vi "Pre Launch Init.vi"(11 "VG-VNA_GUI in":refnum<class "VG-VNA_GUI.lvclass">) -> (0 "error out":errorcluster, 3 "VG-VNA_GUI out":refnum<class "VG-VNA_GUI.lvclass">)   [LabVIEW 2020, in "VG-VNA_GUI.lvlib" / "VG-VNA_GUI.lvclass"]
doc: "(<B>Filename</B>: Actor Framework.lvlib:Actor.lvclass:Pre Launch Init.vi)\n\nDefines behavior that occurs after the Launch Nested Actor method is invoked but before the actor's Actor Core method begins running.\n\nBy default, this method does nothing. A descendant class may override it to define behavior."
uses:
  VG-VNA_GUI.lvclass
  hardware_manager/VHM-VNA_Hardware_Manager/VHM-VNA_Hardware_Manager/VHM-connection_status.ctl
  data_handler/VDH-VNA_data_handler/VDH-VNA_data_handler/VDH-calibration_status.ctl
  data_handler/VDH-VNA_data_handler/VDH-VNA_data_handler/VDH-SOLT_calib_Status.ctl
  data_handler/VDH-VNA_data_handler/VDH-VNA_data_handler/VDH-Calibration_prosess.ctl
  data_handler/VDH-VNA_data_handler/VDH-VNA_data_handler/VDH-Calibration_enum.ctl
  classes/vna-drivers/liteVNA/VD-settings_status.ctl
  VG-graph_data.ctl
  VG-VNA_GUI.lvclass/VG-VNA_GUI.ctl
  <vilib>/ActorFramework/Actor/Actor.lvclass
  classes/vna-drivers/liteVNA/VD-LV-LiteVNA.lvclass
  data_handler/VDH-VNA_data_handler/VDH-VNA_data_handler/VDH-VNA_data_handler.lvclass
  hardware_manager/VHM-VNA_Hardware_Manager/VHM-VNA_Hardware_Manager/VHM-VNA_Hardware_Manager.lvclass
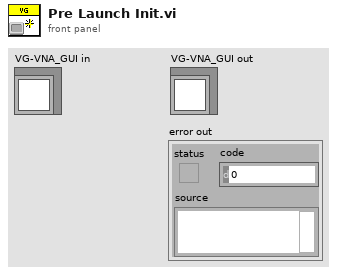
[diagram p1: front panel]
types:
  T1 = typedef "VHM-VNA_Hardware_Manager.lvlib/VHM-VNA_Hardware_Manager.lvclass/VHM-connection_status.ctl" = cluster{"Connected?":bool, "Status":string}
  T2 = typedef "VDH-VNA_data_handler.lvlib/VDH-VNA_data_handler.lvclass/VDH-calibration_status.ctl" = cluster{"Calib Status":T3, "Calibrated?":bool, "Permativity?":bool, "Progress":T4}
  T3 = typedef "VDH-VNA_data_handler.lvlib/VDH-VNA_data_handler.lvclass/VDH-SOLT_calib_Status.ctl" = cluster{"Short":bool, "Open":bool, "Load":bool, "Through":bool}
  T4 = typedef "VDH-VNA_data_handler.lvlib/VDH-VNA_data_handler.lvclass/VDH-Calibration_prosess.ctl" = cluster{"Progress":bool, "current":T5, "samples to get":u8}
  T5 = typedef "VDH-VNA_data_handler.lvlib/VDH-VNA_data_handler.lvclass/VDH-Calibration_enum.ctl" = enum16{"Non", "Short", "Open", "Load", "Through", "Permativity"}
  T6 = typedef "VD-LV-LiteVNA.lvclass/VD-settings_status.ctl" = cluster{"Start [Hz]":u64, "Span [Hz]":u64, "Stop [Mhz]":u64, "Number of points #":u16, "Sample Average #":u16}
  T7 = typedef "VG-VNA_GUI.lvlib/VG-VNA_GUI.lvclass/VG-graph_data.ctl" = cluster{u64[], dbl[]}[]
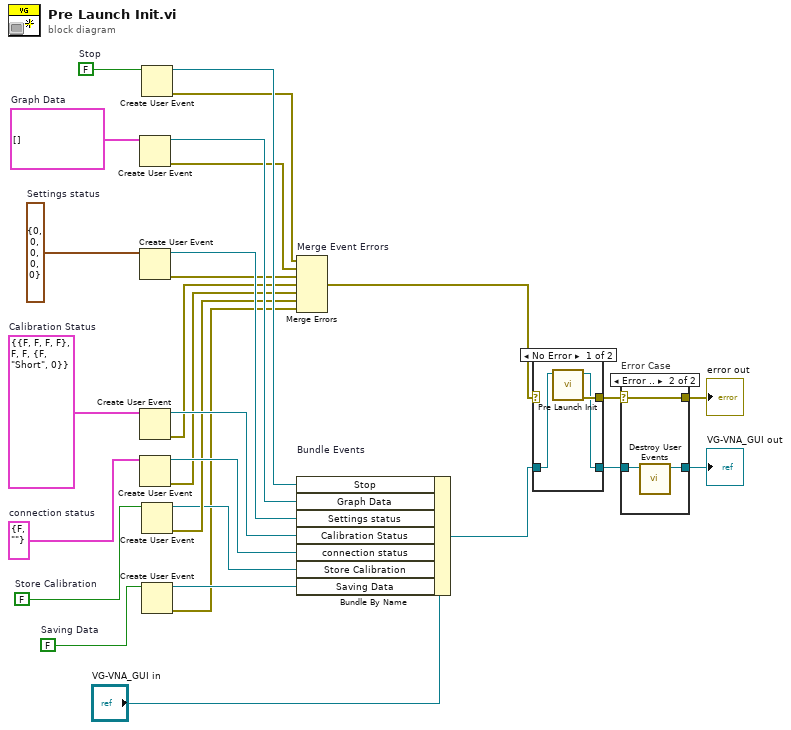
[diagram p0: block diagram]
diagram:
  w3 = FALSE  # Saving Data
  w6 = FALSE  # Store Calibration
  w9 = T1 {"Connected?"=FALSE, "Status"=""}  # connection status
  w12 = T2 {"Calib Status"={"Short"=FALSE, "Open"=FALSE, "Load"=FALSE, "Through"=FALSE}, "Calibrated?"=FALSE, "Permativity?"=FALSE, "Progress"={"Progress"=FALSE, "current"=enum."Short", "samples to get"=0}}  # Calibration Status
  w15 = T6 {"Start [Hz]"=0, "Span [Hz]"=0, "Stop [Mhz]"=0, "Number of points #"=0, "Sample Average #"=0}  # Settings status
  w23 = T7 []  # Graph Data
  w24 = FALSE  # Stop
  n1 = Create User Event(user event datatype=w23) -> (user event=w21:refnum<user-event>, error out=w16:errorcluster)  [unwired: 1 in]
  n2 = Create User Event(user event datatype=w15) -> (user event=w14:refnum<user-event>, error out=w13:errorcluster)  [unwired: 1 in]
  n3 = Create User Event(user event datatype=w12) -> (user event=w11:refnum<user-event>, error out=w10:errorcluster)  [unwired: 1 in]
  n4 = Create User Event(user event datatype=w9) -> (user event=w8:refnum<user-event>, error out=w7:errorcluster)  [unwired: 1 in]
  n5 = Create User Event(user event datatype=w24) -> (user event=w22:refnum<user-event>, error out=w17:errorcluster)  [unwired: 1 in]
  n6 = Create User Event(user event datatype=w6) -> (user event=w4:refnum<user-event>, error out=w5:errorcluster)  [unwired: 1 in]
  n7 = Create User Event(user event datatype=w3) -> (user event=w2:refnum<user-event>, error out=w1:errorcluster)  [unwired: 1 in]
  n8 = Merge Errors "Merge Event Errors"(w17, w16, w13, w10, w7, w5, w1) -> (w27:errorcluster)
  n9 = Bundle By Name "Bundle Events"(cluster="VG-VNA_GUI in", "Stop"=w22, "Graph Data"=w21, "Settings status"=w14, "Calibration Status"=w11, "connection status"=w8, "Store Calibration"=w4, "Saving Data"=w2) -> (w25:refnum<class "VG-VNA_GUI.lvclass">)
  n10 = case shown="No Error" w27 {
    selector: w27 -> [_ w33]
    tunnel: w25 -> [w31 w32]
    tunnel: [w30 w33] -> w26
    tunnel: [w29 w32] -> w20
    frame No Error {
      n11 = call-parent "Pre Launch Init.vi"("Actor in"=w31) -> ("error out"=w30:errorcluster, "Actor out"=w29:refnum<class "VG-VNA_GUI.lvclass">)  [unwired: 9 in]
    }
    frame Error {
    }
  }
  n12 = case "Error Case" shown="Error .." w26 {
    selector: w26 -> [w35 w36]
    tunnel: w20 -> [w34 w38]
    tunnel: [w34 w37] -> w19
    tunnel: [w35 w36] -> w18
    frame No Error {
    }
    frame Error {
      n13 = call "Destroy User Events.vi"("VG-VNA_GUI in"=w38) -> ("VG-VNA_GUI out"=w37:refnum<class "VG-VNA_GUI.lvclass">)  [unwired: 10 in]
    }
  }
  "error out" <- w18
  "VG-VNA_GUI out" <- w19
